vi "getDevice.vi"(8 "error in (no error)":errorcluster, 11 "BasicRemote in":refnum<class "BasicRemote.lvclass">) -> (0 "error out":errorcluster, 2 "Device.lvclass":refnum<class "Device.lvclass">, 3 "BasicRemote out":refnum<class "BasicRemote.lvclass">)   [LabVIEW 2017, in "BasicRemote.lvclass"]
uses:
  BasicRemote.lvclass
  Device Class/Device.lvclass
  BasicRemote.lvclass/BasicRemote.ctl
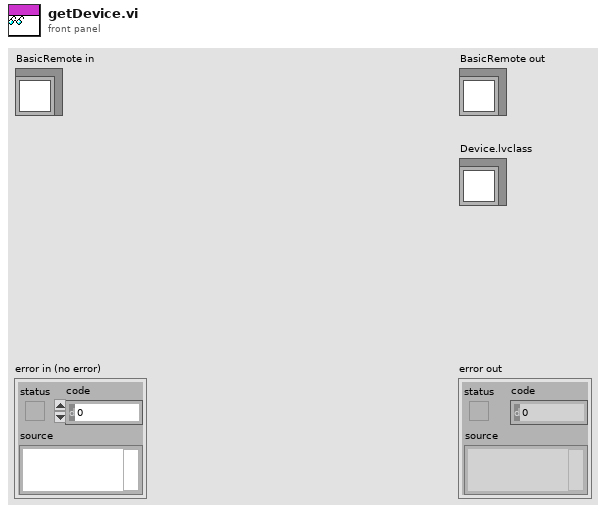
[diagram p1: front panel]
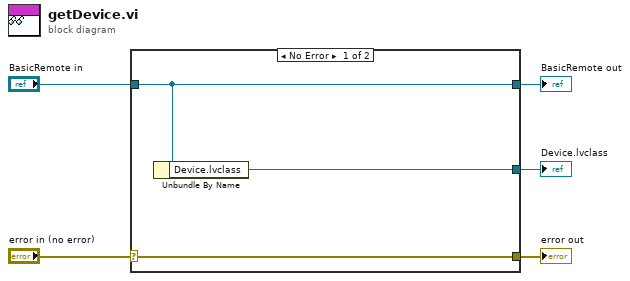
[diagram p0: block diagram]
diagram:
  n1 = case shown="No Error" "error in (no error)" {
    selector: "error in (no error)" -> [w8 w9]
    tunnel: [w8 w9] -> w4
    tunnel: [w7 w10] -> w2
    tunnel: "BasicRemote in" -> [w7 w10]
    tunnel: [w6 _] -> w1
    frame No Error {
      n2 = Unbundle By Name(w7) -> ("Device.lvclass"=w6:refnum<class "Device.lvclass">)
    }
    frame Error {
    }
  }
  "error out" <- w4
  "BasicRemote out" <- w2
  "Device.lvclass" <- w1
